vi "Planta_303_ver 8 Final.vi"() -> ()   [LabVIEW 2014]
uses:
  <vilib>/measure/NI_MABase.lvlib
  <vilib>/addons/System Identification/NI_SysID.lvlib
panel:
  in  "Upsampling Factor":i32=2
  in  "polynomial order":i32=31 caption="Polynomial Order" max=512
  in  "samples":i64=128 caption="Samples"
  out "Gráfico Saída":dynamicdata(graph)
  in  "Duty cycle (%)":dbl=50.0 format="%0.2f"
  out "Tanque":dbl(slide) scale=0.0..300.0
  in  "Escolha o Sinal":string(combo)
  out "Gráfico Entrada":dbl[](graph)
  in  "Amplitude   %":dbl=1.0 caption="Amplitude"
  in  "Frequency":dbl=10.1
  in  "Offset  %":dbl caption="Offset"
  in  "?":u32(colorbox)
  # "DEGRAU"
  # "ENTRADAS"
  # "PRBS"
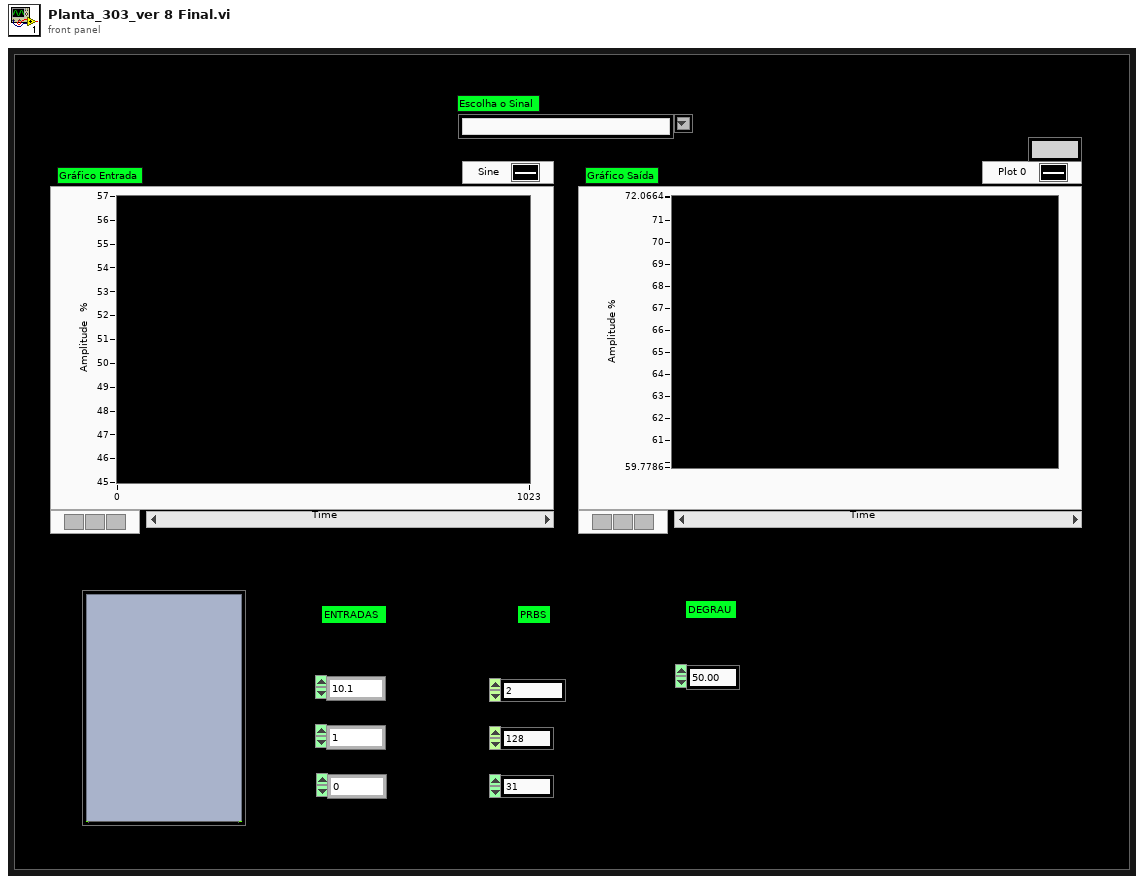
[diagram p1: front panel]
types:
  T1 = enum16{"Sine Wave", "Triangle Wave", "Square Wave", "Sawtooth Wave"}
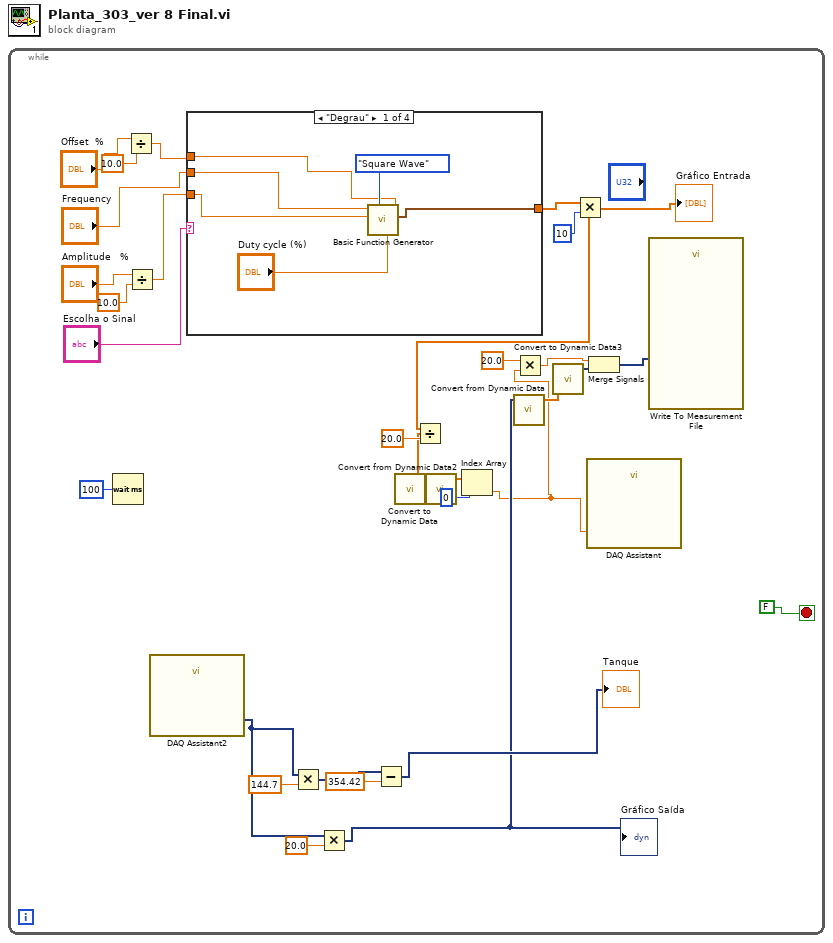
[diagram p0: block diagram]
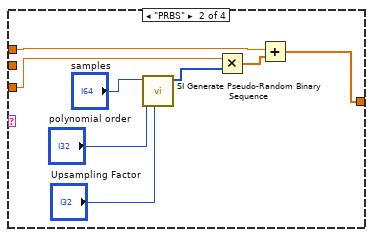
[diagram p2: hidden frame]
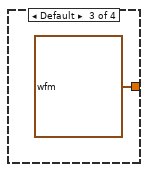
[diagram p3: hidden frame]
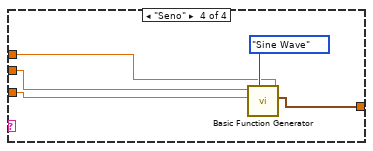
[diagram p4: hidden frame]
diagram:
  n1 = while {
    stop <- FALSE stop-if-true
    n2 = Wait (ms)(milliseconds to wait=u32 100) -> ()  [unwired: 1 out]
    n3 = Divide(x="Offset  %", y=10.0) -> (x/y=w4:dbl)
    n4 = Divide(x="Amplitude   %", y=10.0) -> (x/y=w2:dbl)
    n5 = call "DAQ Assistant2"() -> ("data"=w16:dynamicdata)  [unwired: 17 in, 2 out]
    n6 = case shown="\"Degrau\"" "Escolha o Sinal" {
      tunnel: w4 -> [w36 w43 _ w50]
      tunnel: "Frequency" -> [w35 _ _ w49]
      tunnel: w2 -> [w34 w44 _ w48]
      tunnel: [w33 w41 waveform(dbl) {"t0"=timestamp(0 s since 1904-01-01), "dt"=1.0, "Y"=[]} ("signal out") w47] -> w12
      frame "Degrau" {
        n7 = call <vilib>:"Basic Function Generator.vi"("offset"=w36, "square wave duty cycle (%)"="Duty cycle (%)", "signal type"=T1."Square Wave", "amplitude"=w34, "frequency"=w35) -> ("signal out"=w33:waveform(dbl))  [unwired: 4 in, 2 out]
      }
      frame "PRBS" {
        n8 = call <vilib>:"SI Generate Pseudo-Random Binary Sequence.vi"("upsampling factor"="Upsampling Factor", "polynomial order"="polynomial order", "samples"="samples") -> ("PRBS"=w45:u8[])  [unwired: 8 in]
        n9 = Multiply(x=w44, y=w45) -> (x*y=w42:dbl[])
        n10 = Add(x=w43, y=w42) -> (x+y=w41:dbl[])
      }
      frame Default {
      }
      frame "Seno" {
        n11 = call <vilib>:"Basic Function Generator.vi"("offset"=w50, "signal type"=T1."Sine Wave", "amplitude"=w48, "frequency"=w49) -> ("signal out"=w47:waveform(dbl))  [unwired: 5 in, 2 out]
      }
    }
    n12 = Multiply(x=w16, y=144.7) -> (x*y=w23:dynamicdata)
    n13 = Multiply(x=w16, y=20.0) -> (x*y=w15:dynamicdata)
    "Gráfico Saída" <- w15
    n14 = Subtract(x=w23, y=354.42) -> (x-y=→"Tanque":dynamicdata)
    n15 = call "Convert from Dynamic Data"("Dynamic Data Type"=w15) -> ("Array"=w18:dbl[])  [unwired: 3 in]
    n16 = call "Convert to Dynamic Data3"("Array"=w18) -> ("Dynamic Data Type"=w17:dynamicdata)  [unwired: 3 in]
    n17 = Multiply(x=w12, y=10) -> (x*y=w13:dbl[])
    "Gráfico Entrada" <- w13
    n18 = Divide(x=w13, y=20.0) -> (x/y=w25:dbl[])
    n19 = call "Convert to Dynamic Data"("Array"=w25) -> ("Dynamic Data Type"=w20:dynamicdata)  [unwired: 3 in]
    n20 = call "Convert from Dynamic Data2"("Dynamic Data Type"=w20) -> ("Array"=w27:dbl[])  [unwired: 3 in]
    n21 = Index Array "Index Array"(array=w27, index=0) -> (element=w9:dbl)
    n22 = Multiply(x=20.0, y=w9) -> (x*y=w8:dbl)
    n23 = call "DAQ Assistant"("data"=w9) -> ()  [unwired: 17 in, 2 out]
    n24 = Merge Signals(w8, w17) -> (w19:dynamicdata)
    n25 = call "Write To Measurement File"("Signals"=w19) -> ()  [unwired: 16 in, 3 out]
  }
